vi "EnvCoverTest.vi"() -> ()   [LabVIEW 2016]
panel:
  out "Open":bool
  out "Closed":bool
  in  "CoverState":enum16{"In", "Moving", "Out", "Wait"}(ring)
  in  "stop":bool
  out "Ready?":bool=TRUE
  out "error out":errorcluster={"status"=FALSE, "code"=-1950679034, "source"="Shared Variable in EnvCoverRT.vi->MainRT.vi<APPEND>\nThis error or warning occurred while reading the following Shared Variable:\n\\\\fem-rt\\RT-Variables\\CoverState\n\\\\172.29.46.109\\RT-Variables\\CoverState"}
  out "Status out":enum16{"In", "Moving", "Out", "Wait"}(ring)
  in  "error in (no error)":errorcluster
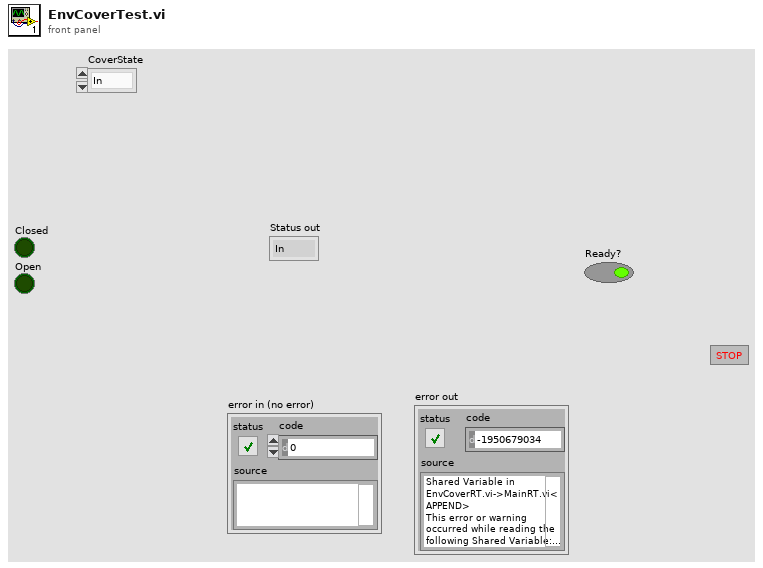
[diagram p1: front panel]
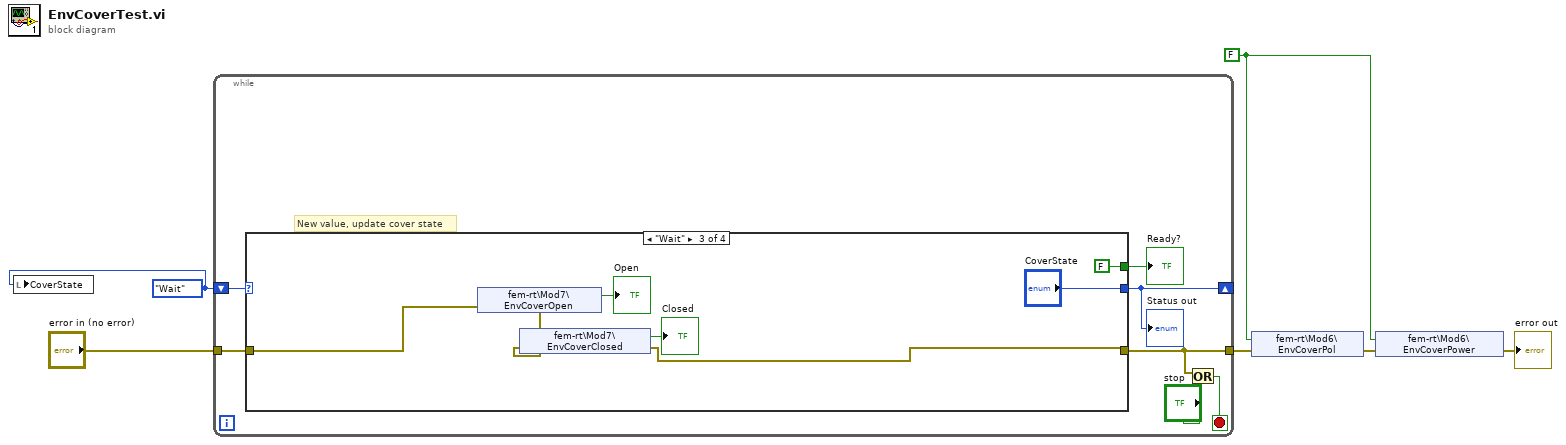
[diagram p0: block diagram]
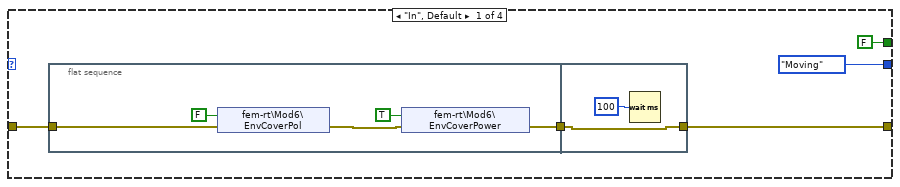
[diagram p2: hidden frame]
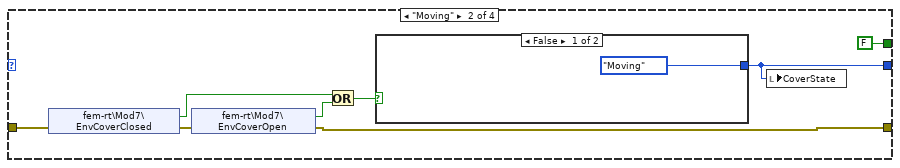
[diagram p3: hidden frame]
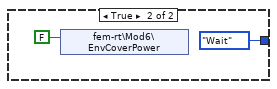
[diagram p4: hidden frame]
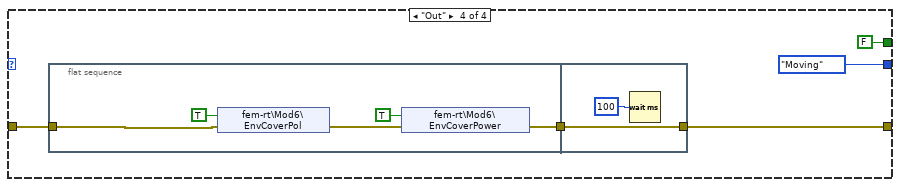
[diagram p5: hidden frame]
diagram:
  w2 = FALSE ("EnvCoverPol")
  w1 = enum16{"In", "Moving", "Out", "Wait"}."Wait" ("Status")
  n1 = local write "CoverState"(w1) -> ()
  n2 = while {
    tunnel: "error in (no error)" -> [w10]
    tunnel: [w9] -> w3
    shift-right: [w12] -> _
    shift-left: w1 -> [w11]
    stop <- w7 stop-if-true
    # "New value, update cover state"
    n3 = case shown="\"Wait\"" w11 {
      tunnel: [enum16{"In", "Moving", "Out", "Wait"}."Moving" ("Status") w26 "CoverState" enum16{"In", "Moving", "Out", "Wait"}."Moving" ("Status")] -> w12
      tunnel: [w18 w27 w37 w47] -> w9
      tunnel: w10 -> [w17 w29 w39 w48]
      tunnel: [FALSE FALSE FALSE FALSE] -> w13
      frame "In", Default {
        n4 = flat-sequence {
          tunnel: w17 -> [w20]
          tunnel: [w21] -> w15
          tunnel: [w25] -> w18
          tunnel: w15 -> [w25]
          frame #0 {
            n5 = shared-variable "fem-rt\\Mod6\\EnvCoverPol"(FALSE ("EnvCoverPol"), error in=w20) -> (error out=w22:errorcluster)
            n6 = shared-variable "fem-rt\\Mod6\\EnvCoverPower"(TRUE, error in=w22) -> (error out=w21:errorcluster)
          }
          frame #1 {
            n7 = Wait (ms)(milliseconds to wait=u32 100) -> ()  [unwired: 1 out]
          }
        }
      }
      frame "Moving" {
        n8 = shared-variable "fem-rt\\Mod7\\EnvCoverClosed"(error in=w29) -> (w32:bool, error out=w28:errorcluster)
        n9 = shared-variable "fem-rt\\Mod7\\EnvCoverOpen"(error in=w28) -> (w31:bool, error out=w27:errorcluster)
        n10 = Or(x=w32, y=w31) -> (x .or. y?=w30:bool)
        n11 = case shown="False" w30 {
          tunnel: [enum16{"In", "Moving", "Out", "Wait"}."Moving" ("Status") enum16{"In", "Moving", "Out", "Wait"}."Wait" ("Status")] -> w26
          frame False {
          }
          frame True {
            n12 = shared-variable "fem-rt\\Mod6\\EnvCoverPower"(FALSE) -> ()  [unwired: 1 in, 1 out]
          }
        }
        n13 = local write "CoverState"(w26) -> ()
      }
      frame "Wait" {
        n14 = shared-variable "fem-rt\\Mod7\\EnvCoverOpen"(error in=w39) -> (→"Open":bool, error out=w38:errorcluster)
        n15 = shared-variable "fem-rt\\Mod7\\EnvCoverClosed"(error in=w38) -> (→"Closed":bool, error out=w37:errorcluster)
      }
      frame "Out" {
        n16 = flat-sequence {
          tunnel: w48 -> [w52]
          tunnel: [w51] -> w45
          tunnel: [w55] -> w47
          tunnel: w45 -> [w55]
          frame #0 {
            n17 = shared-variable "fem-rt\\Mod6\\EnvCoverPol"(TRUE ("EnvCoverPol"), error in=w52) -> (error out=w53:errorcluster)
            n18 = shared-variable "fem-rt\\Mod6\\EnvCoverPower"(TRUE ("EnvCoverPower"), error in=w53) -> (error out=w51:errorcluster)
          }
          frame #1 {
            n19 = Wait (ms)(milliseconds to wait=u32 100) -> ()  [unwired: 1 out]
          }
        }
      }
    }
    "Status out" <- w12
    "Ready?" <- w13
    n20 = Or(x=w9, y="stop") -> (x .or. y?=w7:bool)
  }
  n21 = shared-variable "fem-rt\\Mod6\\EnvCoverPol"(w2, error in=w3) -> (error out=w5:errorcluster)
  n22 = shared-variable "fem-rt\\Mod6\\EnvCoverPower"(w2, error in=w5) -> (error out=→"error out":errorcluster)
